vi "Teleop.vi"(10 "Match Info":T1={"Autonomous Elapsed Seconds"=0.0, "TeleOp Elapsed Seconds"=0.0, "Disabled Elapsed Seconds"=0.0, "Visited Autonomous"=FALSE, "Visited TeleOp"=FALSE, "Visited Disabled"=FALSE, "Autonomous Settings"={"Autonomous Style"=enum."Independent", "VI Refnum"=refnum}}, 11 "Call Context":T2) -> ()   [LabVIEW 2016]
doc: "This VI is called for each TeleOp packet received from the DS where the robot is not disabled. It is often used to read from the joysticks and update I/O or to update setpoints for timed control loops. It should complete and return within 20 milliseconds or it may miss DS packets."
uses:
  <vilib>/Rock Robotics/WPI/DriverStation/WPI_DriverStationDerivedRobotMode.ctl
  <vilib>/Rock Robotics/WPI/DriverStation/WPI_DriverStationMatch Info.ctl
  <vilib>/Rock Robotics/Network Tables/NT Read Numeric Array.vi
  <vilib>/Rock Robotics/Network Tables/NT Write String.vi
  Drive/Drive Globals.vi
  Rotation/Rotation Globals.vi
  Intake/Intake Globals.vi
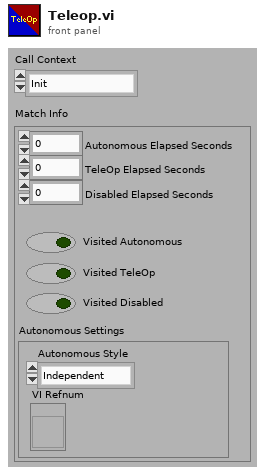
[diagram p1: front panel]
types:
  T1 = typedef "WPI_DriverStationMatch Info.ctl" = cluster{"Autonomous Elapsed Seconds":dbl, "TeleOp Elapsed Seconds":dbl, "Disabled Elapsed Seconds":dbl, "Visited Autonomous":bool, "Visited TeleOp":bool, "Visited Disabled":bool, "Autonomous Settings":cluster{"Autonomous Style":enum16{"Iterative", "Independent"}, "VI Refnum":refnum<vi>}}
  T2 = typedef "WPI_DriverStationDerivedRobotMode.ctl" = enum16{"Init", "Execute", "Stop"}
  T3 = typedef "Robot Controls.ctl" = cluster{"Right Joystick Trigger":bool, "Right Joystick Thumb Button":bool, "Right Joystick Button 3":bool, "Right Joystick Button 4":bool, "Right Joystick Button 5":bool, "Right Joystick Button 7":bool, "Right Joystick Button 8":bool, "Right Joystick Button 9":bool, "Right Joystick Button 10":bool, "Right Joystick Button 11":bool, "Right Joystick Left - Right":dbl, "Right Joystick Up-Down":dbl, "Right Joystick Twist":dbl, "Right Joystick Throttle":dbl, "Right Joystick Button 6":bool, "Right Joystick Button 12":bool, "Left  Joystick Trigger":bool, "Left Joystick Button 2":bool, "Left Joystick Button 3":bool, "Left Joystick Left - Right":dbl, "Left Joystick Up-Down":dbl, "Left Joystick Throttle ":dbl, "Left Joystick Button 4":bool, "Left Joystick Button 5":bool, "Left Joystick Button 6":bool, "Left Joystick Button 7":bool, "Left Joystick Button 8":bool, "Left Joystick Button 9":bool, "Left Joystick Button 10":bool, "Left Joystick Button 11":bool, "Left Joystick Button 12":bool, "POV":dbl}
  T4 = typedef "Rotation Notifier.ctl" = cluster{"Up":bool, "Down":bool, "Rotation Control List":T5, "Control Down":bool, "Manual":bool, "Parameter 1":dbl, "Parameter 2":dbl}
  T5 = typedef "Rotation Control Type.ctl" = enum16{"No Op", "Up", "Down", "Control Up", "Control Down"}
  T6 = typedef "Drive Notifier.ctl" = cluster{"Parameter 1":dbl, "Parameter 2":dbl, "Parameter 3":dbl, "Drive Control List":T7, "Parameter 4":dbl, "Gear Angle":dbl, "Parameter 6":dbl, "Parameter 7":dbl, "Parameter 8":dbl, "Parameter 9":dbl, "Robotcentric":bool, "Reset Gyro":bool, "Reset Wheels":bool, "Turn to Gear Left":bool, "Turn to Gear Center":bool, "Turn to Gear Right":bool, "Half Power":bool}
  T7 = typedef "Drive Control Type.ctl" = enum16{"No Op", "Fieldcentric", "Robotcentric", "Reset Wheel Position", "Reset Gyro Value", "Turn to Angle", "Drive For Time"}
  T8 = typedef "Intake Notifier.ctl" = cluster{"In":bool, "Out":bool, "Intake Control List":T9, "Parameter 1":dbl, "Parameter 2":dbl}
  T9 = typedef "Intake Control Type.ctl" = enum16{"No Op", "In", "Out"}
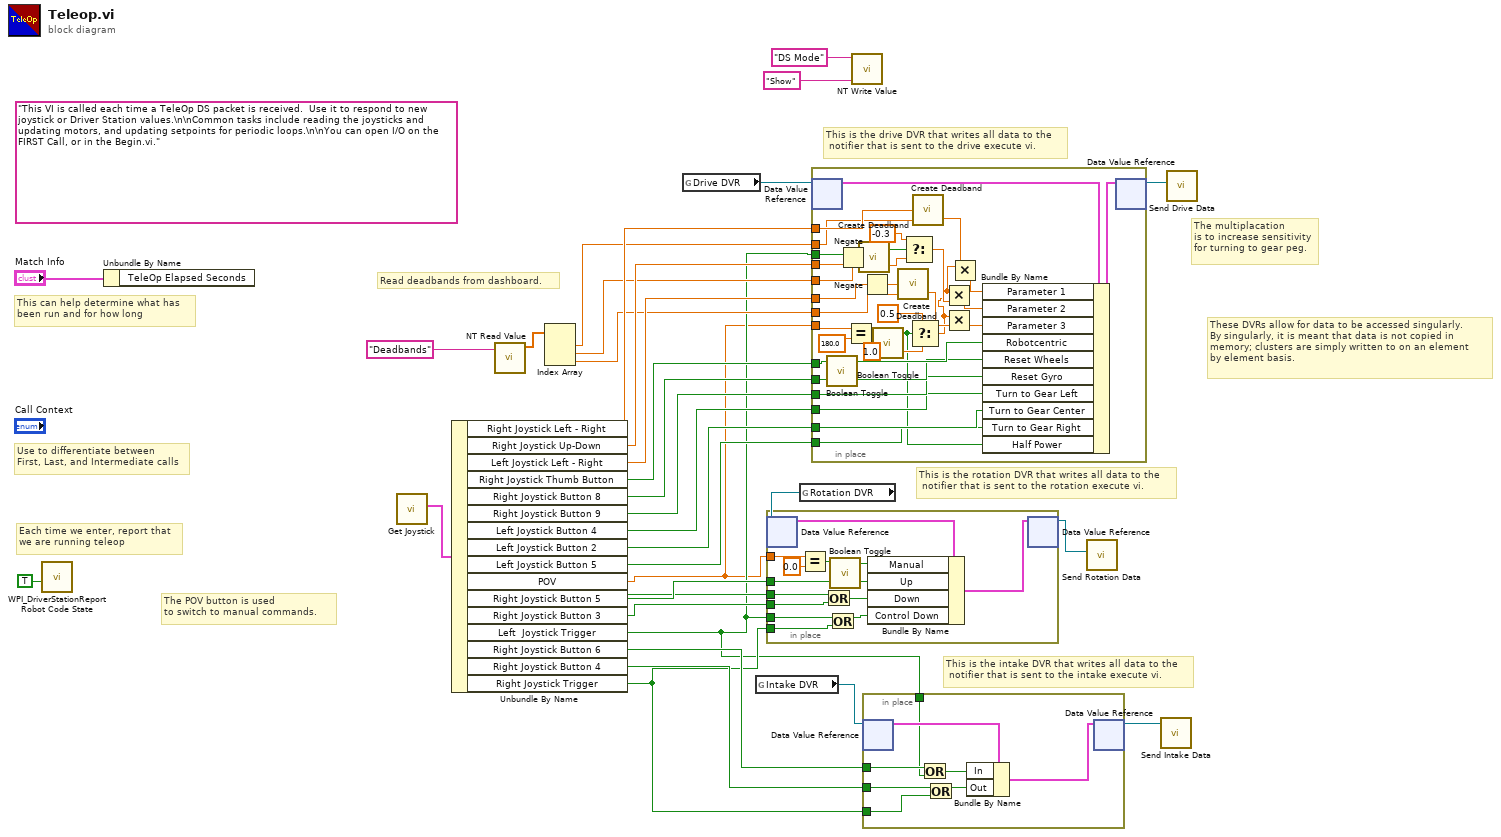
[diagram p0: block diagram]
diagram:
  (unwired) "This VI is called each time a TeleOp DS packet is received.  Use it to respond to new joystick or Driver Station values.\n\nCommon tasks include reading the joysticks and updating motors, and updating setpoints for periodic loops.\n\nYou can open I/O on the FIRST Call, or in the Begin.vi."
  # "The multiplacation\nis to increase sensitivity\nfor turning to gear peg."
  # "The POV button is used\nto switch to manual commands."
  # "This is the intake DVR that writes all data to the\n notifier that is sent to the intake execute vi."
  # "This is the rotation DVR that writes all data to the\n notifier that is sent to the rotation execute vi."
  # "This is the drive DVR that writes all data to the\n notifier that is sent to the drive execute vi."
  # "These DVRs allow for data to be accessed singularly.\nBy singularly, it is meant that data is not copied in\nmemory; clusters are simply written to on an element\nby element basis."
  # "Read deadbands from dashboard."
  # "Each time we enter, report that\nwe are running teleop"
  # "Use to differentiate between\nFirst, Last, and Intermediate calls"
  # "This can help determine what has\nbeen run and for how long"
  n1 = call <vilib>:"WPI_DriverStationReport Robot Code State.vi"("TeleOp"=TRUE ("Autonomous")) -> ()  [unwired: 10 in, 1 out]
  n2 = Unbundle By Name("Match Info") -> ()  [unwired: 1 out]
  n3 = call "Get Joystick.vi"() -> ("Robot Controls"=w24:T3)  [unwired: 11 in]
  n4 = Unbundle By Name(w24) -> ("Right Joystick Left - Right"=w23:dbl, "Right Joystick Up-Down"=w22:dbl, "Left Joystick Left - Right"=w18:dbl, "Right Joystick Thumb Button"=w21:bool, "Right Joystick Button 8"=w20:bool, "Right Joystick Button 9"=w19:bool, "Left Joystick Button 4"=w9:bool, "Left Joystick Button 2"=w8:bool, "Left Joystick Button 5"=w7:bool, "POV"=w1:dbl, "Right Joystick Button 5"=w17:bool, "Right Joystick Button 3"=w6:bool, "Left  Joystick Trigger"=w4:bool, "Right Joystick Button 6"=w16:bool, "Right Joystick Button 4"=w15:bool, "Right Joystick Trigger"=w5:bool)
  n5 = call-poly <vilib>:"NT Read Value.vi"("Name"="Deadbands") -> ("Numeric Array"=w13:dbl[])  [unwired: 9 in, 1 out]
  n6 = Index Array(array=w13) -> (element #1=w12:dbl, element #2=w11:dbl, element #3=w10:dbl)  [unwired: 3 in]
  n7 = global read "Drive Globals.vi" "Drive DVR"() -> (w30:refnum<data-value>)
  n8 = global read "Intake Globals.vi" "Intake DVR"() -> (w26:refnum<data-value>)
  n9 = global read "Rotation Globals.vi" "Rotation DVR"() -> (w28:refnum<data-value>)
  n10 = in-place {
    in-place-border: w17 -> [w43]
    in-place-border: w6 -> [w39]
    in-place-border: w4 -> [w42]
    in-place-border: w6 -> [w40]
    in-place-border: w5 -> [w37]
    in-place-border: w1 -> [w33]
    n11 = in-place-dvr #1(w28) -> (w45:T4)  [unwired: 1 out]
    n12 = Equal?(x=w33, y=0.0) -> (x = y?=w35:bool)
    n13 = Or(x=w39, y=w40) -> (x .or. y?=w41:bool)
    n14 = Or(x=w42, y=w37) -> (x .or. y?=w38:bool)
    n15 = call "Boolean Toggle.vi"("Input"=w35) -> ("Output"=w34:bool)  [unwired: 26 in]
    n16 = Bundle By Name(cluster=w45, "Manual"=w34, "Up"=w43, "Down"=w41, "Control Down"=w38) -> (w44:T4)
    n17 = in-place-dvr #1(w44) -> (w27:refnum<data-value>)  [unwired: 1 out]
  }
  n18 = in-place {
    in-place-border: w22 -> [w72]
    in-place-border: w21 -> [w75]
    in-place-border: w23 -> [w71]
    in-place-border: w20 -> [w74]
    in-place-border: w19 -> [w73]
    in-place-border: w18 -> [w70]
    in-place-border: w12 -> [w68]
    in-place-border: w11 -> [w67]
    in-place-border: w10 -> [w66]
    in-place-border: w9 -> [w65]
    in-place-border: w8 -> [w64]
    in-place-border: w7 -> [w63]
    in-place-border: w4 -> [w56]
    in-place-border: w1 -> [w51]
    n19 = in-place-dvr #2(w30) -> (w78:T6)  [unwired: 1 out]
    n20 = call "Boolean Toggle.vi"("Input"=w75) -> ("Output"=w76:bool)  [unwired: 26 in]
    n21 = Negate(x=w72) -> (-x=w62:dbl)
    n22 = Equal?(x=w51, y=180.0) -> (x = y?=w53:bool)
    n23 = call "Create Deadband.vi"("Input Deadband"=w67, "Input"=w62) -> ("Output"=w58:dbl)  [unwired: 2 in]
    n24 = Negate(x=w70) -> (-x=w61:dbl)
    n25 = call "Boolean Toggle.vi"("Input"=w53) -> ("Output"=w46:bool)  [unwired: 26 in]
    n26 = call "Create Deadband.vi"("Input Deadband"=w66, "Input"=w61) -> ("Output"=w69:dbl)  [unwired: 2 in]
    n27 = Select(t=-0.3, s=w56, f=w58) -> (s? t:f=w59:dbl)
    n28 = Select(t=0.5, s=w46, f=1.0) -> (s? t:f=w47:dbl)
    n29 = call "Create Deadband.vi"("Input Deadband"=w68, "Input"=w71) -> ("Output"=w60:dbl)  [unwired: 2 in]
    n30 = Multiply(x=w47, y=w59) -> (x*y=w49:dbl)
    n31 = Multiply(x=w47, y=w69) -> (x*y=w48:dbl)
    n32 = Multiply(x=w47, y=w60) -> (x*y=w50:dbl)
    n33 = Bundle By Name(cluster=w78, "Parameter 1"=w50, "Parameter 2"=w49, "Parameter 3"=w48, "Robotcentric"=w76, "Reset Wheels"=w74, "Reset Gyro"=w73, "Turn to Gear Left"=w65, "Turn to Gear Center"=w64, "Turn to Gear Right"=w63, "Half Power"=w46) -> (w77:T6)
    n34 = in-place-dvr #2(w77) -> (w29:refnum<data-value>)  [unwired: 1 out]
  }
  n35 = call-poly <vilib>:"NT Write Value.vi"("String"="Show", "Name"="DS Mode") -> ()  [unwired: 9 in, 1 out]
  n36 = in-place {
    in-place-border: w16 -> [w84]
    in-place-border: w15 -> [w83]
    in-place-border: w4 -> [w82]
    in-place-border: w5 -> [w79]
    n37 = in-place-dvr #3(w26) -> (w86:T8)  [unwired: 1 out]
    n38 = Or(x=w84, y=w82) -> (x .or. y?=w81:bool)
    n39 = Or(x=w83, y=w79) -> (x .or. y?=w80:bool)
    n40 = Bundle By Name(cluster=w86, "In"=w81, "Out"=w80) -> (w85:T8)
    n41 = in-place-dvr #3(w85) -> (w25:refnum<data-value>)  [unwired: 1 out]
  }
  n42 = call "Send Rotation Data.vi"("DVR In"=w27) -> ()  [unwired: 11 in]
  n43 = call "Send Intake Data.vi"("DVR In"=w25) -> ()  [unwired: 11 in]
  n44 = call "Send Drive Data.vi"("DVR In"=w29) -> ()  [unwired: 10 in]
